vi "calcContZStackParams.vi"(0 "zPosInit (mm)":dbl, 5 "zPosFin (mm)":dbl=10.0, 7 "zIncrement (mm)":dbl=1.0, 9 "Exposure time (s)":dbl=0.1, 11 "opticalSectionThickness(mm)":dbl=0.05) -> (6 "new zPosInit (mm)":dbl, 8 "new zPosFin (mm)":dbl, 10 "fine axial vel (mm/s)":dbl=10.0, 15 "acqDelay (ms)":u32=10)   [LabVIEW 2015]
panel:
  in  "minAcqVel":dbl=0.0001
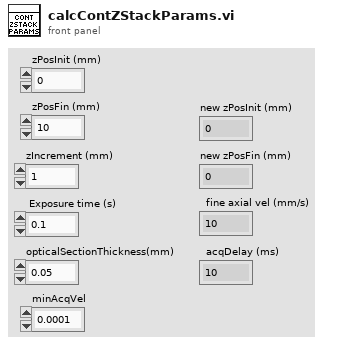
[diagram p1: front panel]
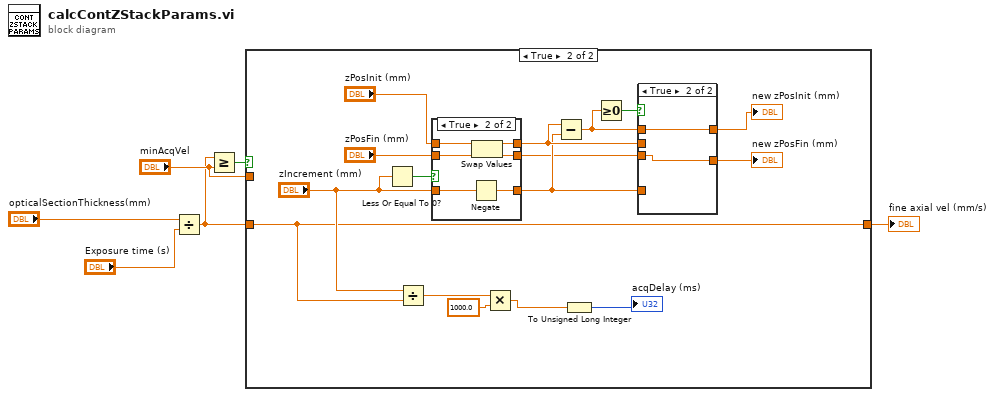
[diagram p0: block diagram]
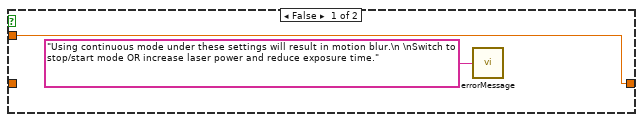
[diagram p2: hidden frame]
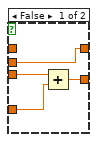
[diagram p3: hidden frame]
diagram:
  n1 = Divide(x="opticalSectionThickness(mm)", y="Exposure time (s)") -> (x/y=w2:dbl)
  n2 = Greater Or Equal?(x=w2, y="minAcqVel") -> (x >= y?=w5:bool)
  n3 = case shown="True" w5 {
    tunnel: [w7 w10] -> w3
    tunnel: "minAcqVel" -> [w7 _]
    tunnel: w2 -> [_ w10]
    frame False {
      n4 = call "errorMessage.vi"("messageText"="Using continuous mode under these settings will result in motion blur.\n \nSwitch to stop/start mode OR increase laser power and reduce exposure time.") -> ()  [unwired: 3 out]
    }
    frame True {
      n5 = Less Or Equal To 0?(x="zIncrement (mm)") -> (x <= 0?=w24:bool)
      n6 = Divide(x="zIncrement (mm)", y=w10) -> (x/y=w12:dbl)
      n7 = case shown="True" w24 {
        tunnel: "zIncrement (mm)" -> [w33 w39]
        tunnel: [w33 w38] -> w16
        tunnel: "zPosInit (mm)" -> [w32 w37]
        tunnel: "zPosFin (mm)" -> [w31 w36]
        tunnel: [w32 w35] -> w20
        tunnel: [w31 w34] -> w15
        frame False {
        }
        frame True {
          n8 = Negate(x=w39) -> (-x=w38:dbl)
          n9 = Swap Values(12:w37, 14:w36) -> (1:w35:dbl, 3:w34:dbl)  [unwired: 1 in]
        }
      }
      n10 = Multiply(x=w12, y=1000.0) -> (x*y=w14:dbl)
      n11 = Subtract(x=w20, y=w16) -> (x-y=w19:dbl)
      n12 = To Unsigned Long Integer(number=w14) -> (unsigned 32bit integer=→"acqDelay (ms)":u32)
      n13 = Greater Or Equal To 0?(x=w19) -> (x >= 0?=w21:bool)
      n14 = case shown="True" w21 {
        tunnel: w20 -> [w28 _]
        tunnel: [w28 w30] -> w18
        tunnel: w19 -> [_ w30]
        tunnel: [w27 w29] -> w17
        tunnel: w16 -> [w26 _]
        tunnel: w15 -> [w25 w29]
        frame False {
          n15 = Add(x=w25, y=w26) -> (x+y=w27:dbl)
        }
        frame True {
        }
      }
      "new zPosFin (mm)" <- w17
      "new zPosInit (mm)" <- w18
    }
  }
  "fine axial vel (mm/s)" <- w3
